vi "Simple MQTT Client.vi"() -> ()   [LabVIEW 2020]
uses:
  <vilib>/LabVIEW Open Source Project/MQTT Client/Client class/Client.lvclass/Client.ctl
  <vilib>/LabVIEW Open Source Project/MQTT Connection/MQTT_Base/Base Class/MQTT_Base.lvclass/MQTT_Base.ctl
  <vilib>/LabVIEW Open Source Project/MQTT TCP Connection/MQTT_TCP/Connection/TCPConnection.lvclass
  C:/Program Files (x86)/National Instruments/LabVIEW 2020/vi.lib/LabVIEW Open Source Project/MQTT Connection/MQTT_Connection/Connection/Connection.lvclass
  <vilib>/LabVIEW Open Source Project/MQTT Client/Client class/Client.lvclass
  C:/Program Files (x86)/National Instruments/LabVIEW 2020/vi.lib/LabVIEW Open Source Project/MQTT Connection/MQTT_Base/Base Class/MQTT_Base.lvclass
  <vilib>/LabVIEW Open Source Project/MQTT Control Packets/Control Packets/PUBLISH/PUBLISH.lvclass
  <vilib>/LabVIEW Open Source Project/MQTT Connection/MQTT_Base/Base Class/MQTT_Base.lvclass
panel:
  out "data":string[](array[string])
  out "Unsuback":bool
  out "Suback":bool
  in  "Subscribe":bool
  in  "Connection":bool
  in  "Stop Client":bool
  out "last error":errorcluster
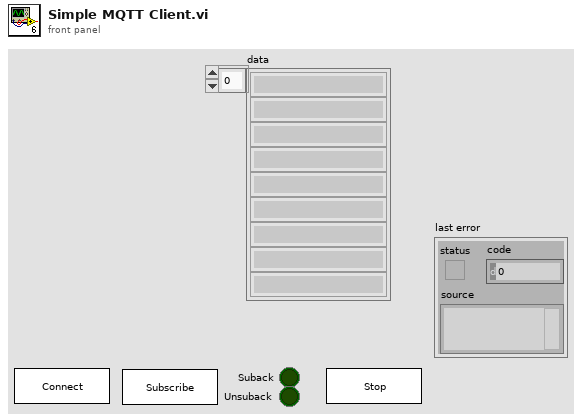
[diagram p1: front panel]
types:
  T1 = typedef "MQTT Client.lvlib/Client.lvclass/Public Events -- cluster.ctl" = cluster{"Connection Status":refnum<user-event>, "Connected":refnum<user-event>, "Application Message":refnum<user-event>}
  T2 = typedef "MQTT Base.lvlib/MQTT_Base.lvclass/Public Events -- cluster.ctl" = cluster{"Stop Event":refnum<user-event>, "Error Event":refnum<user-event>, "Inbound Message":refnum<user-event>}
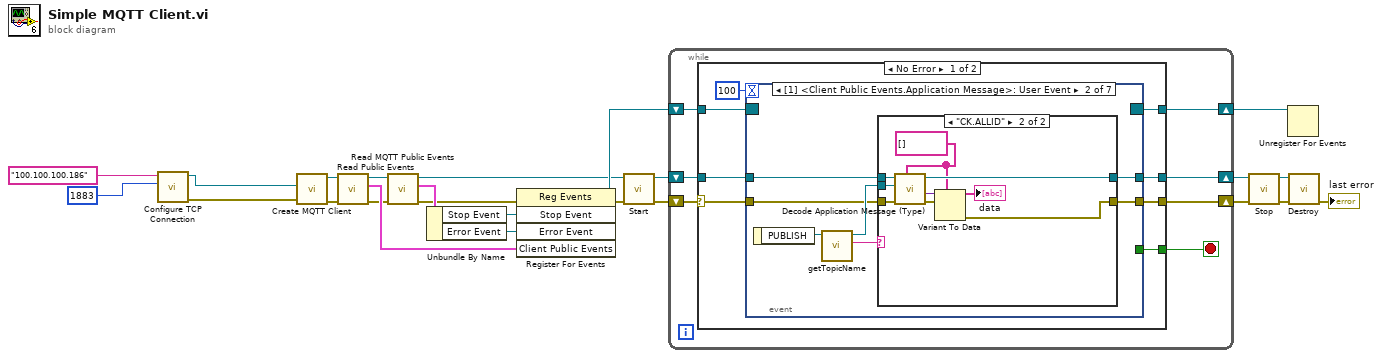
[diagram p0: block diagram]
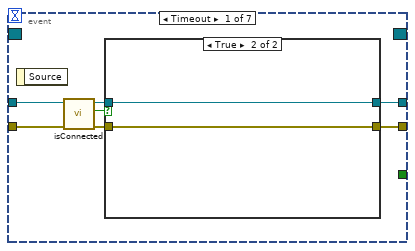
[diagram p2: hidden frame]
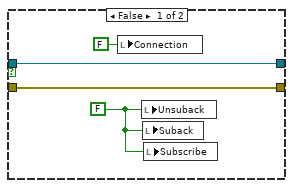
[diagram p3: hidden frame]
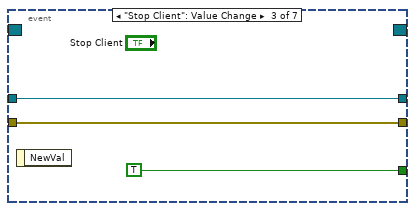
[diagram p5: hidden frame]
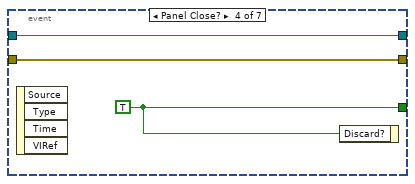
[diagram p6: hidden frame]
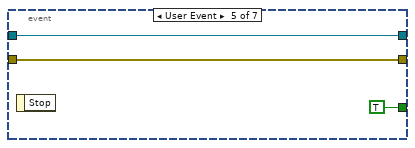
[diagram p7: hidden frame]
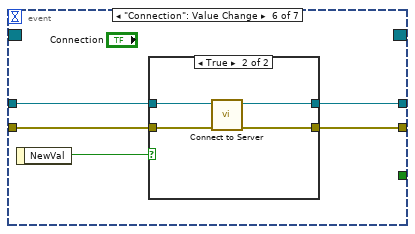
[diagram p8: hidden frame]
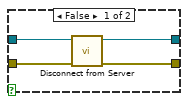
[diagram p9: hidden frame]
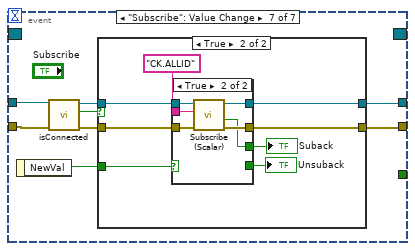
[diagram p10: hidden frame]
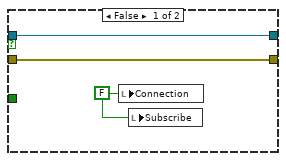
[diagram p11: hidden frame]
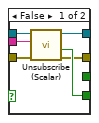
[diagram p12: hidden frame]
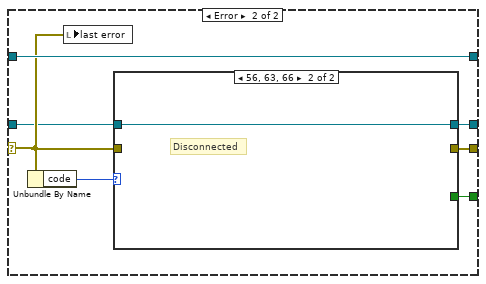
[diagram p13: hidden frame]
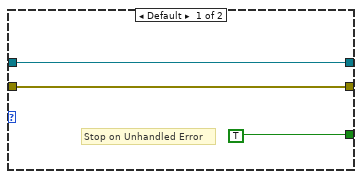
[diagram p14: hidden frame]
diagram:
  n1 = call <vilib>:"Configure TCP Connection.vi"("remote port (80)"=u16 1883, "address (localhost)"="100.100.100.186") -> ("error out"=w3:errorcluster, "TCPConnection"=w4:refnum<class "TCPConnection.lvclass">)  [unwired: 8 in]
  n2 = call <vilib>:"Create MQTT Client.vi"("error in (no error)"=w3, "Connection Configuration"=w4) -> ("error out"=w7:errorcluster, "Client out"=w5:refnum<class "Client.lvclass">)  [unwired: 8 in]
  n3 = call <vilib>:"Read Public Events.vi"("error in (no error)"=w7, "Client in"=w5) -> ("error out"=w8:errorcluster, "Client Public Events"=w10:T1, "Client out"=w6:refnum<class "Client.lvclass">)  [unwired: 7 in]
  n4 = call <vilib>:"Read MQTT Public Events.vi"("error in (no error)"=w8, "MQTT_Base in"=w6) -> ("error out"=w9:errorcluster, "MQTT Public Events"=w17:T2, "MQTT_Base out"=w12:refnum<class "Client.lvclass">)  [unwired: 7 in]
  n5 = Unbundle By Name(w17) -> ("Stop Event"=w15:refnum<user-event>, "Error Event"=w16:refnum<user-event>)
  n6 = register-events(error in=w9, w15, w16, w10) -> (reference out=w13:refnum<event-registration>, error out=w11:errorcluster)  [unwired: 1 in]
  n7 = call <vilib>:"Start.vi"("error in (no error)"=w11, "MQTT_Base in"=w12) -> ("error out"=w23:errorcluster, "MQTT_Base out"=w22:refnum<class "Client.lvclass">)  [unwired: 7 in, 1 out]
  n8 = while {
    shift-right: [w30] -> w14
    shift-left: w13 -> [w31]
    shift-right: [w27] -> w19
    shift-left: w22 -> [w28]
    shift-right: [w29] -> w21
    shift-left: w23 -> [w25]
    stop <- w26 stop-if-true
    n9 = case shown="No Error" w25 {
      selector: w25 -> [w32 w127]
      tunnel: w31 -> [w39 w130]
      tunnel: [w38 w130] -> w30
      tunnel: [w37 w125] -> w29
      tunnel: w28 -> [w35 w126]
      tunnel: [w34 w129] -> w27
      tunnel: [w33 w124] -> w26
      frame No Error {
        n10 = event shown="[1] <Client Public Events.Application Message>: User Event" {
          selector: w39 -> [_ _ _ _ _ _ _]
          dyn-events: [_ _ _ _ _ _ _] -> w38
          timeout: 100 -> [_ _ _ _ _ _ _]
          tunnel: w32 -> [w42 w56 w72 w74 w79 w80 w98]
          tunnel: [w45 w53 w72 w74 w79 w81 w99] -> w37
          tunnel: [_ _ TRUE w76 TRUE _ _] -> w33
          tunnel: w35 -> [w44 w57 w73 w75 w77 w84 w97]
          tunnel: [w46 w55 w73 w75 w77 w82 w100] -> w34
          event Timeout {
            n11 = event-data() -> ()  [unwired: 1 in, 1 out]
            n12 = call <vilib>:"isConnected.vi"("error in (no error)"=w42, "Client in"=w44) -> ("error out"=w41:errorcluster, "connected"=w40:bool, "Client out"=w43:refnum<class "Client.lvclass">)  [unwired: 7 in]
            n13 = case shown="True" w40 {
              tunnel: [w50 w52] -> w46
              tunnel: [w49 w51] -> w45
              tunnel: w43 -> [w50 w52]
              tunnel: w41 -> [w49 w51]
              frame False {
                w48 = FALSE
                n14 = local write "Connection"(FALSE ("Connection")) -> ()
                n15 = local write "Unsuback"(w48) -> ()
                n16 = local write "Suback"(w48) -> ()
                n17 = local write "Subscribe"(w48) -> ()
              }
              frame True {
              }
            }
          }
          event User Event {
            n18 = event-data() -> ("PUBLISH"=w59:refnum<class "PUBLISH.lvclass">)  [unwired: 1 in]
            n19 = call <vilib>:"getTopicName.vi"("PUBLISH in"=w59) -> ("Topic"=w54:string, "PUBLISH out"=w58:refnum<class "PUBLISH.lvclass">)  [unwired: 8 in, 1 out]
            n20 = case shown="\"CK.ALLID\"" w54 {
              tunnel: w58 -> [_ w64]
              tunnel: w57 -> [w61 w69]
              tunnel: w56 -> [w60 w67]
              tunnel: [w61 w68] -> w55
              tunnel: [w60 w70] -> w53
              frame Default {
              }
              frame "CK.ALLID" {
                w63 = string[] []
                n21 = call <vilib>:"Decode Application Message (Type).vi"("Type"=w63, "error in (no error)"=w67, "PUBLISH"=w64, "Client in"=w69) -> ("error out"=w66:errorcluster, "Payload"=w65:variant, "Client out"=w68:refnum<class "Client.lvclass">)  [unwired: 4 in, 1 out]
                n22 = Variant To Data(error in=w66, type=w63, Variant=w65) -> (data=→"data":string[], error out=w70:errorcluster)
              }
            }
          }
          event "Stop Client": Value Change {
            n23 = event-data() -> ()  [unwired: 1 in, 1 out]
          }
          event Panel Close? {
            w76 = TRUE
            n24 = event-data() -> ()  [unwired: 1 in, 4 out]
            n25 = event-data("Discard?"=w76) -> ()  [unwired: 1 in, 1 out]
          }
          event User Event {
            n26 = event-data() -> ()  [unwired: 1 in, 1 out]
          }
          event "Connection": Value Change {
            n27 = event-data() -> ("NewVal"=w83:bool)  [unwired: 1 in]
            n28 = case shown="True" w83 {
              tunnel: w84 -> [w88 w92]
              tunnel: [w87 w89] -> w82
              tunnel: [w86 w90] -> w81
              tunnel: w80 -> [w85 w91]
              frame False {
                n29 = call <vilib>:"Disconnect from Server.vi"("error in (no error)"=w85, "Client in"=w88) -> ("error out"=w86:errorcluster, "Client out"=w87:refnum<class "Client.lvclass">)  [unwired: 7 in, 1 out]
              }
              frame True {
                n30 = call <vilib>:"Connect to Server.vi"("error in (no error)"=w91, "Client in"=w92) -> ("error out"=w90:errorcluster, "Client out"=w89:refnum<class "Client.lvclass">)  [unwired: 6 in, 2 out]
              }
            }
          }
          event "Subscribe": Value Change {
            n31 = event-data() -> ("NewVal"=w93:bool)  [unwired: 1 in]
            n32 = call <vilib>:"isConnected.vi"("error in (no error)"=w98, "Client in"=w97) -> ("error out"=w95:errorcluster, "connected"=w94:bool, "Client out"=w96:refnum<class "Client.lvclass">)  [unwired: 7 in]
            n33 = case shown="True" w94 {
              tunnel: [w103 w111] -> w100
              tunnel: [w102 w110] -> w99
              tunnel: w96 -> [w103 w109]
              tunnel: w95 -> [w102 w108]
              tunnel: w93 -> [_ w106]
              frame False {
                w101 = FALSE ("Connection")
                n34 = local write "Connection"(w101) -> ()
                n35 = local write "Subscribe"(w101) -> ()
              }
              frame True {
                n36 = case shown="True" w106 {
                  tunnel: [w112 w120] -> w111
                  tunnel: [w113 w119] -> w110
                  tunnel: w109 -> [w117 w123]
                  tunnel: w108 -> [w116 w122]
                  tunnel: "CK.ALLID" ("Topic Name (empty: Payload name)") -> [w115 w121]
                  tunnel: [_ w118] -> w105
                  tunnel: [w114 _] -> w104
                  frame False {
                    n37 = call <vilib>:"Unsubscribe (Scalar).vi"("error in (no error)"=w116, "Topic Filter"=w115, "Client in"=w117) -> ("error out"=w113:errorcluster, "Ack"=w114:bool, "Client out"=w112:refnum<class "Client.lvclass">)  [unwired: 6 in]
                  }
                  frame True {
                    n38 = call <vilib>:"Subscribe (Scalar).vi"("error in (no error)"=w122, "Topic Filter"=w121, "Client in"=w123) -> ("error out"=w119:errorcluster, "Ack"=w118:bool, "Client out"=w120:refnum<class "Client.lvclass">)  [unwired: 6 in]
                  }
                }
                "Unsuback" <- w104
                "Suback" <- w105
              }
            }
          }
        }
      }
      frame Error {
        n39 = Unbundle By Name(w127) -> ("code"=w128:i32)
        n40 = local write "last error"(w127) -> ()
        n41 = case shown="56, 63, 66" w128 {
          tunnel: w126 -> [w133 w134]
          tunnel: [w133 w134] -> w129
          tunnel: w127 -> [w132 _]
          tunnel: [w132 _] -> w125
          tunnel: [TRUE _] -> w124
          frame Default {
            # "Stop on Unhandled Error"
          }
          frame 56, 63, 66 {
            # "Disconnected"
          }
        }
      }
    }
  }
  n42 = call <vilib>:"Stop.vi"("error in (no error)"=w21, "MQTT_Base in"=w19) -> ("error out"=w20:errorcluster, "MQTT_Base out"=w18:refnum<class "Client.lvclass">)  [unwired: 7 in, 1 out]
  n43 = Unregister For Events(event registration refnum=w14) -> ()  [unwired: 1 in, 1 out]
  n44 = call <vilib>:"Destroy.vi"("error in (no error)"=w20, "MQTT_Base in"=w18) -> ("error out"=→"last error":errorcluster)  [unwired: 8 in, 1 out]
